vi "Begin.vi"() -> ()   [LabVIEW 2015]
doc: "Called before other user functions, this VI is expected to open initial I/O refnums, load in file data, and do all program initialization. Notice that the <B>error out</B> terminal is simply used for data flow. Wiring it to other structures or subVIs ensures that this VI runs first."
uses:
  <vilib>/Rock Robotics/WPI/DriverStation/WPI_DriverStationRobotMode2.ctl
  <vilib>/Rock Robotics/WPI/Joystick/WPI_JoystickDeviceEnum.ctl
  <vilib>/Rock Robotics/SystemInterfaces/DIO/FPGA_DIOChannel.ctl
  <vilib>/Rock Robotics/WPI/Encoder/WPI_EncoderType.ctl
  <vilib>/Rock Robotics/WPI/CAN/TalonSRX/WPI_CANTalonSRX_APIControlMode.ctl
  <vilib>/Rock Robotics/WPI/CAN/TalonSRX/WPI_CANTalonSRX_APIFeedbackSelect.ctl
  <vilib>/Rock Robotics/SystemInterfaces/DIO/FPGA_DIOPWMChannel.ctl
  Robot Global Data.vi
  <vilib>/Rock Robotics/Network Tables/NT Write String Array.vi
  <vilib>/Rock Robotics/WPI/Counter/WPI_CounterDigitalInputToDigitalSource.vi
  <vilib>/Rock Robotics/WPI/MotorControl/WPI_MotorControlOpenCANTalonSRX.vi
  <vilib>/Rock Robotics/WPI/MotorControl/WPI_MotorControlOpen VictorSP.vi
panel:
  in  "error in":errorcluster
  out "error out":errorcluster
  in  "I 3":dbl
  in  "F 3":dbl=0.01
  in  "D 3":dbl caption="D"
  in  "P 3":dbl=1.0 caption="P"
  in  "Reverse Feedback Sensor 3":bool
  in  "Slave Device Number 3":u8=1 caption="Slave Device Number"
  in  "Encoder Codes Per Rev 3":u16=360
  in  "Master Device Number 3":u8 caption="Master Device Number"
  in  "I 2":dbl
  in  "F 2":dbl=0.01
  in  "D 2":dbl caption="D"
  in  "P 2":dbl=1.0 caption="P"
  in  "Reverse Feedback Sensor 2":bool
  in  "Slave Device Number 2":u8=1 caption="Slave Device Number"
  in  "Encoder Codes Per Rev 2":u16=360
  in  "Master Device Number 2":u8 caption="Master Device Number"
  in  "I":dbl
  in  "F":dbl=0.01
  in  "D":dbl
  in  "P":dbl=1.0
  in  "Reverse Feedback Sensor":bool
  in  "Slave Device Number":u8=1
  in  "Encoder Codes Per Rev":u16=360
  in  "Master Device Number":u8
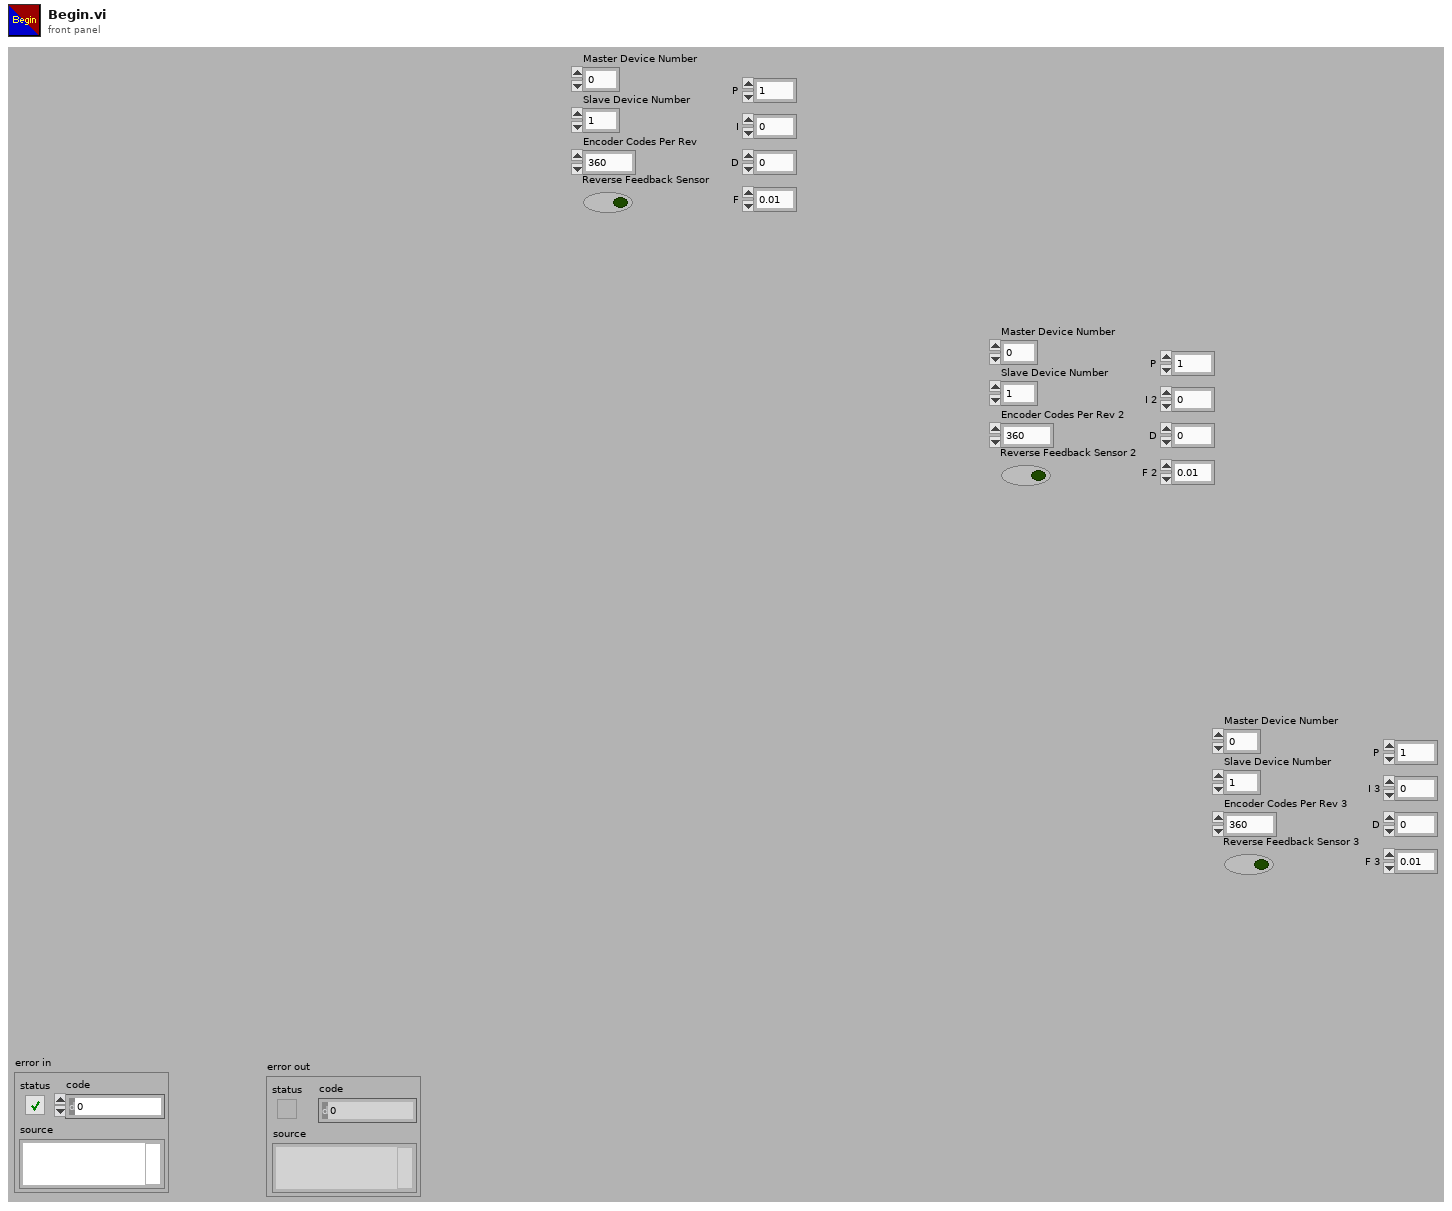
[diagram p1: front panel]
types:
  T1 = typedef "FPGA_DIOPWMChannel.ctl" = enum8{"PWM 0", "PWM 1", "PWM 2", "PWM 3", "PWM 4", "PWM 5", "PWM 6", "PWM 7", "PWM 8", "PWM 9", "PWM MXP 0", "PWM MXP 1", "PWM MXP 2", "PWM MXP 3", "PWM MXP 4", "PWM MXP 5", "PWM MXP 6", "PWM MXP 7", "PWM MXP 8", "PWM MXP 9", "Invalid"}
  T2 = typedef "WPI_EncoderType.ctl" = enum16{"1x", "2x", "4x"}
  T3 = typedef "FPGA_DIOChannel.ctl" = enum8{"DIO 0", "DIO 1", "DIO 2", "DIO 3", "DIO 4", "DIO 5", "DIO 6", "DIO 7", "DIO 8", "DIO 9", "DIO MXP 0", "DIO MXP 1", "DIO MXP 2", "DIO MXP 3", "DIO MXP 4", "DIO MXP 5", "DIO MXP 6", "DIO MXP 7", "DIO MXP 8", "DIO MXP 9", "DIO MXP 10", "DIO MXP 11", "DIO MXP 12", "DIO MXP 13", "DIO MXP 14", "DIO MXP 15", "Invalid"}
  T4 = typedef "WPI_JoystickDeviceEnum.ctl" = enum16{"USB 0", "USB 1", "USB 2", "USB 3", "USB 4", "USB 5"}
  T5 = typedef "WPI_CANTalonSRX_APIControlMode.ctl" = enum8{"Percent VBus", "Speed", "Position", "Slave", "Unchanged / Invalid", "Voltage Compensation", "Current", "Motion Profile"}
  T6 = typedef "WPI_CANTalonSRX_APIFeedbackSelect.ctl" = enum16{"Digital Quadrature Encoder", "Analog Potentiometer", "Analog Encoder", "Count on Quad-A (Rising-Edge)", "Count on Quad-A (Falling-Edge)", "CTR Magnetic Enc (Absolute)", "CTR Magnetic Enc (Relative)", "Pulse Width"}
  T7 = typedef "WPI_DriverStationRobotMode2.ctl" = enum16{"Autonomous Disabled", "Autonomous Enabled", "Teleop Disabled", "Teleop Enabled", "Disconnected", "Finish", "Test Disabled", "Test Enabled", "Emergency Stopped"}
  T8 = typedef "WPI_MotorControlDeviceRef.ctl" = cluster{"DeviceStatus":errorcluster, "Type":T9, "PWM":cluster{"PWM Channel":T1, "DeadBand":T10}, "CAN":cluster{"Device Number":u8, "Control Mode":T11, "Semaphore":T12, "Max Vout":dbl, "TalonSRX Control Mode":T5}, "Invert":bool}
  T9 = typedef "WPI_MotorControlType.ctl" = enum16{"PWM", "CAN", "CANTalonSRX"}
  T10 = typedef "WPI_PWMDeadband.ctl" = cluster{"Name":string, "maxPositivePwm":i32, "minPositivePwm":i32, "centerPwm":i32, "maxNegativePwm":i32, "minNegativePwm":i32, "angularRange":u16}
  T11 = typedef "WPI_CANJaguar_ControlMode.ctl" = enum8{"Percent VBus", "Current", "Speed", "Position", "Voltage"}
  T12 = typedef "Semaphore RefNum" = refnum<k1>
  T13 = typedef "WPI_JoystickDevRef.ctl" = cluster{"Device":T4}
  T14 = typedef "WPI_DigitalInputDevRef.ctl" = cluster{"DevStatus":errorcluster, "DIO Channel":T3}
  T15 = typedef "FPGA_CounterEncoderSourceConvertionLVSourceType.ctl" = cluster{"DevStatus":errorcluster, "AnalogTriggerMode?":bool, "DigitalMode":cluster{"DIO Channel":T16}, "AnalogTriggerMode":cluster{"AnalogTriggerIndex":T17, "OutputType":T18}}
  T16 = typedef "FPGA_DIODigitalSourceChannel.ctl" = enum8{"DIO 0", "DIO 1", "DIO 2", "DIO 3", "DIO 4", "DIO 5", "DIO 6", "DIO 7", "DIO 8", "DIO 9", "DIO MXP 0", "DIO MXP 1", "DIO MXP 2", "DIO MXP 3", "DIO MXP 4", "DIO MXP 5", "DIO MXP 6", "DIO MXP 7", "DIO MXP 8", "DIO MXP 9", "DIO MXP 10", "DIO MXP 11", "DIO MXP 12", "DIO MXP 13", "DIO MXP 14", "DIO MXP 15", "Disabled"}
  T17 = typedef "FPGA_AnalogTriggerIndex.ctl" = enum8{"Trig 0", "Trig 1", "Trig 2", "Trig 3", "Trig 4", "Trig 5", "Trig 6", "Trig 7", "Invalid"}
  T18 = typedef "FPGA_AnalogTriggerOutType.ctl" = enum16{"InWindow", "TriggerState", "Rising", "Falling"}
  T19 = typedef "WPI_EncoderDevRef.ctl" = cluster{"DevStatus":errorcluster, "EncoderIndex":T20, "CounterIndex":T21, "DistancePerCount":dbl, "Decoding Type":T2}
  T20 = typedef "FPGA_EncoderIdx.ctl" = enum8{"Enc 0", "Enc 1", "Enc 2", "Enc 3", "Enc 4", "Enc 5", "Enc 6", "Enc 7", "Invalid"}
  T21 = typedef "FPGA_CounterCtrSystemIndex.ctl" = enum8{"Ctr 0", "Ctr 1", "Ctr 2", "Ctr 3", "Ctr 4", "Ctr 5", "Ctr 6", "Ctr 7", "Invalid"}
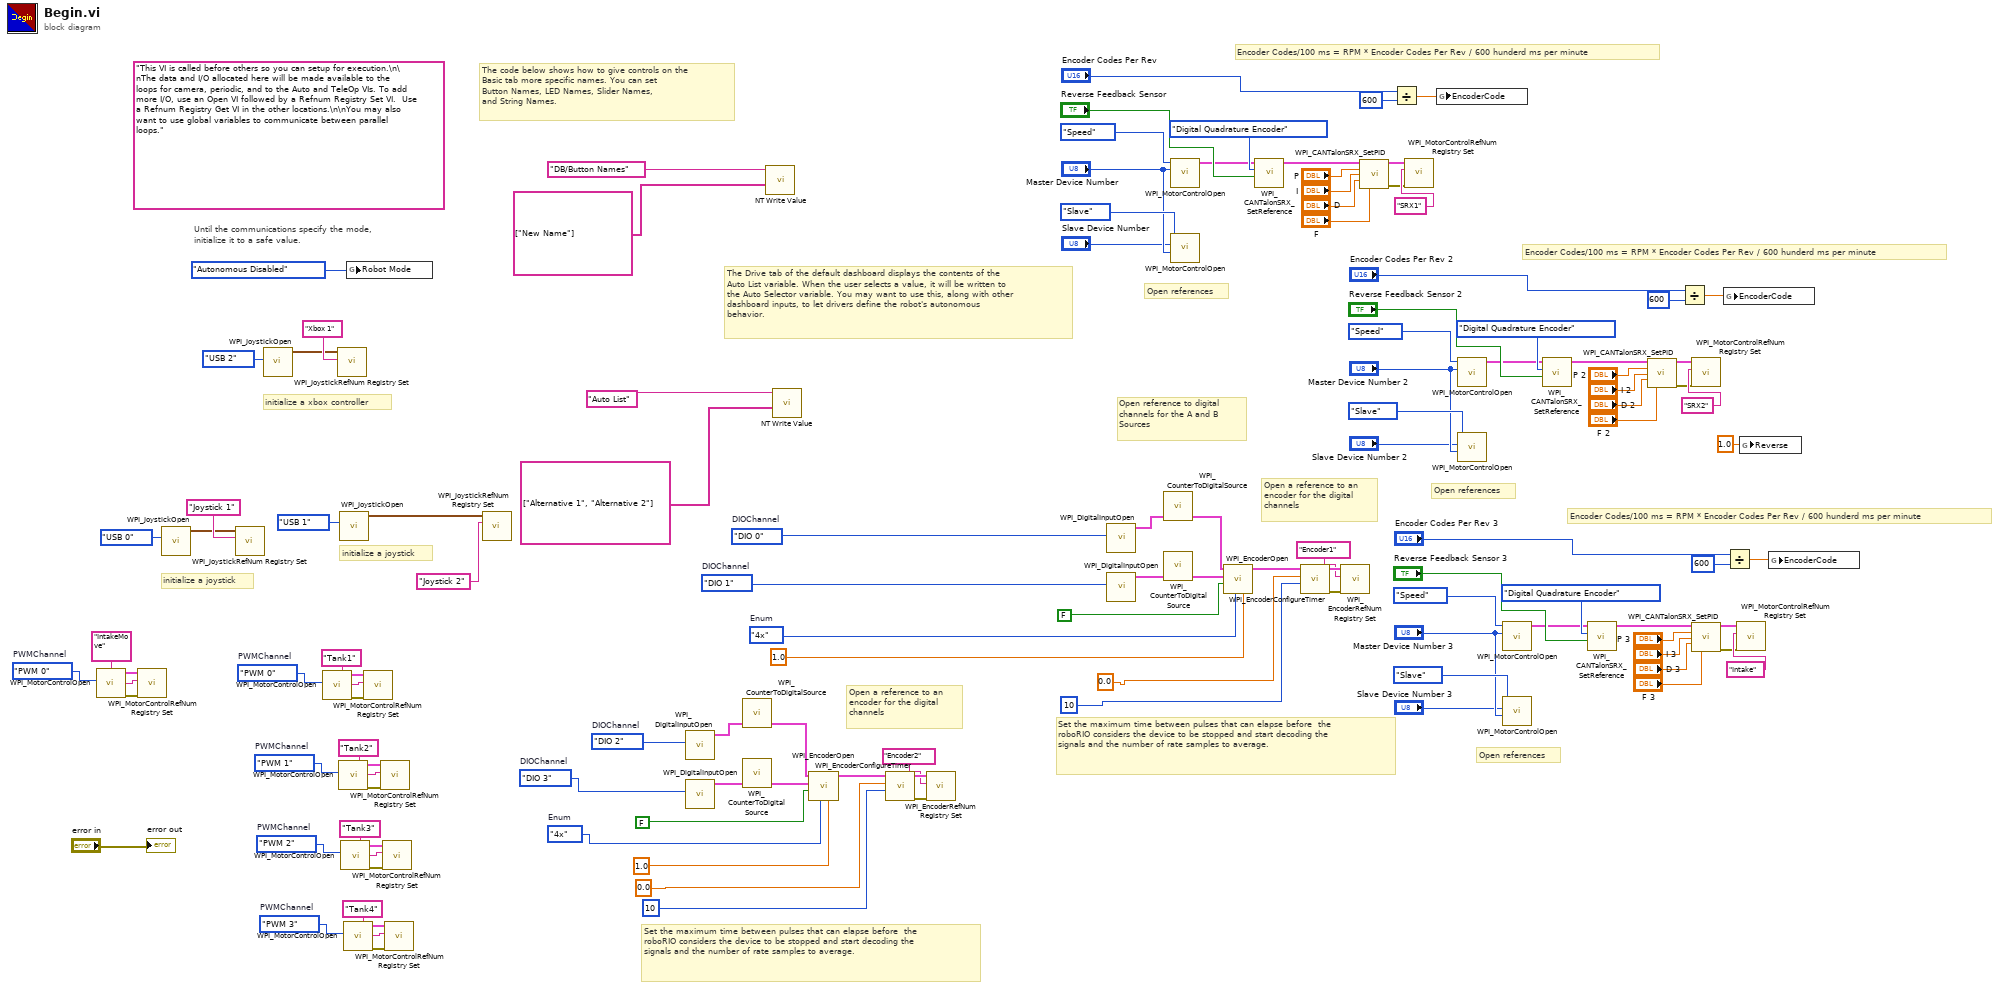
[diagram p0: block diagram]
diagram:
  w2 = FPGA_DIOPWMChannel."PWM 0"  # PWMChannel
  w6 = FPGA_DIOPWMChannel."PWM 3"  # PWMChannel
  w10 = FPGA_DIOPWMChannel."PWM 2"  # PWMChannel
  w14 = FPGA_DIOPWMChannel."PWM 1"  # PWMChannel
  w18 = FPGA_DIOPWMChannel."PWM 0"  # PWMChannel
  w26 = WPI_EncoderType."4x"  # Enum
  w28 = FPGA_DIOChannel."DIO 3"  # DIOChannel
  w29 = FPGA_DIOChannel."DIO 2"  # DIOChannel
  w98 = WPI_EncoderType."4x"  # Enum
  w100 = FPGA_DIOChannel."DIO 1"  # DIOChannel
  w101 = FPGA_DIOChannel."DIO 0"  # DIOChannel
  (unwired) "This VI is called before others so you can setup for execution.\n\nThe data and I/O allocated here will be made available to the loops for camera, periodic, and to the Auto and TeleOp VIs. To add more I/O, use an Open VI followed by a Refnum Registry Set VI.  Use a Refnum Registry Get VI in the other locations.\n\nYou may also want to use global variables to communicate between parallel loops."
  # "Set the maximum time between pulses that can elapse before  the roboRIO considers the device to be stopped and start decoding the signals and the number of rate samples to average."
  # "Open a reference to an\nencoder for the digital \nchannels"
  # "initialize a xbox controller"
  # "Encoder Codes/100 ms = RPM * Encoder Codes Per Rev / 600 hunderd ms per minute"
  # "Open references"
  # "Encoder Codes/100 ms = RPM * Encoder Codes Per Rev / 600 hunderd ms per minute"
  # "Open references"
  # "Encoder Codes/100 ms = RPM * Encoder Codes Per Rev / 600 hunderd ms per minute"
  # "Open references"
  # "The Drive tab of the default dashboard displays the contents of the\nAuto List variable. When the user selects a value, it will be written to\nthe Auto Selector variable. You may want to use this, along with other\ndashboard inputs, to let drivers define the robot's autonomous\nbehavior."
  # "Set the maximum time between pulses that can elapse before  the roboRIO considers the device to be stopped and start decoding the signals and the number of rate samples to average."
  # "Open a reference to an\nencoder for the digital \nchannels"
  # "Open reference to digital \nchannels for the A and B\nSources"
  # "initialize a joystick"
  # "initialize a joystick"
  # "The code below shows how to give controls on the\nBasic tab more specific names. You can set\nButton Names, LED Names, Slider Names,\nand String Names."
  # "Until the communications specify the mode,\ninitialize it to a safe value."
  n1 = call-poly <vilib>:"WPI_MotorControlOpen.vi"("PWM Channel"=w2) -> ("error out"=w5:errorcluster, "MotorControlDeviceRef"=w4:T8)  [unwired: 9 in]
  n2 = call <vilib>:"WPI_MotorControlRefNum Registry Set.vi"("error in (no error)"=w5, "refnum name"="IntakeMove", "MotorControlDevRef"=w4) -> ()  [unwired: 7 in, 2 out]
  n3 = call <vilib>:"WPI_JoystickOpen.vi"("JoystickDevice"=WPI_JoystickDeviceEnum."USB 0") -> ("JoystickDevRef"=w114:T13)  [unwired: 10 in]
  n4 = call <vilib>:"WPI_JoystickRefNum Registry Set.vi"("refnum name"="Joystick 1", "JoystickDevRef"=w114) -> ()  [unwired: 8 in, 2 out]
  n5 = call <vilib>:"WPI_JoystickOpen.vi"("JoystickDevice"=WPI_JoystickDeviceEnum."USB 2") -> ("JoystickDevRef"=w39:T13)  [unwired: 10 in]
  n6 = call-poly <vilib>:"WPI_MotorControlOpen.vi"("PWM Channel"=w18) -> ("error out"=w21:errorcluster, "MotorControlDeviceRef"=w20:T8)  [unwired: 9 in]
  n7 = call <vilib>:"WPI_JoystickRefNum Registry Set.vi"("refnum name"="Xbox 1", "JoystickDevRef"=w39) -> ()  [unwired: 8 in, 2 out]
  n8 = call-poly <vilib>:"WPI_MotorControlOpen.vi"("PWM Channel"=w14) -> ("error out"=w17:errorcluster, "MotorControlDeviceRef"=w16:T8)  [unwired: 9 in]
  n9 = call <vilib>:"WPI_JoystickOpen.vi"("JoystickDevice"=WPI_JoystickDeviceEnum."USB 1") -> ("JoystickDevRef"=w111:T13)  [unwired: 10 in]
  n10 = call-poly <vilib>:"WPI_MotorControlOpen.vi"("PWM Channel"=w10) -> ("error out"=w13:errorcluster, "MotorControlDeviceRef"=w12:T8)  [unwired: 9 in]
  n11 = call-poly <vilib>:"WPI_MotorControlOpen.vi"("PWM Channel"=w6) -> ("error out"=w9:errorcluster, "MotorControlDeviceRef"=w8:T8)  [unwired: 9 in]
  n12 = global write "Robot Global Data.vi" "Robot Mode"(WPI_DriverStationRobotMode2."Autonomous Disabled" ("Robot Mode")) -> ()
  n13 = call <vilib>:"WPI_MotorControlRefNum Registry Set.vi"("error in (no error)"=w21, "refnum name"="Tank1", "MotorControlDevRef"=w20) -> ()  [unwired: 7 in, 2 out]
  n14 = call <vilib>:"WPI_MotorControlRefNum Registry Set.vi"("error in (no error)"=w17, "refnum name"="Tank2", "MotorControlDevRef"=w16) -> ()  [unwired: 7 in, 2 out]
  n15 = call <vilib>:"WPI_MotorControlRefNum Registry Set.vi"("error in (no error)"=w13, "refnum name"="Tank3", "MotorControlDevRef"=w12) -> ()  [unwired: 7 in, 2 out]
  n16 = call <vilib>:"WPI_MotorControlRefNum Registry Set.vi"("error in (no error)"=w9, "refnum name"="Tank4", "MotorControlDevRef"=w8) -> ()  [unwired: 7 in, 2 out]
  n17 = call <vilib>:"WPI_JoystickRefNum Registry Set.vi"("refnum name"="Joystick 2", "JoystickDevRef"=w111) -> ()  [unwired: 8 in, 2 out]
  n18 = call <vilib>:"WPI_DigitalInputOpen.vi"("DIO Channel"=w29) -> ("DigitalInputDevRef"=w35:T14)  [unwired: 1 in, 9 out]
  n19 = call <vilib>:"WPI_DigitalInputOpen.vi"("DIO Channel"=w28) -> ("DigitalInputDevRef"=w36:T14)  [unwired: 1 in, 9 out]
  n20 = call-poly <vilib>:"WPI_CounterToDigitalSource.vi"("DigitalInputDevRef"=w35) -> ("Digital Source"=w34:T15)  [unwired: 6 out]
  n21 = call-poly <vilib>:"WPI_CounterToDigitalSource.vi"("DigitalInputDevRef"=w36) -> ("Digital Source"=w37:T15)  [unwired: 6 out]
  n22 = call-poly <vilib>:"NT Write Value.vi"("String Array"=string[] ["New Name"], "Name"="DB/Button Names") -> ()  [unwired: 9 in, 1 out]
  n23 = call-poly <vilib>:"NT Write Value.vi"("String Array"=string[] ["Alternative 1", "Alternative 2"], "Name"="Auto List") -> ()  [unwired: 9 in, 1 out]
  n24 = call <vilib>:"WPI_EncoderOpen.vi"("DistancePerCount"=1.0, "Decoding Type"=w26, "Invert Direction (False)"=FALSE, "BSource"=w37, "ASource"=w34) -> ("EncoderDevRef"=w33:T19)  [unwired: 3 in, 3 out]
  n25 = call <vilib>:"WPI_EncoderConfigureTimer.vi"("Number Samples to Average"=10, "Minimum Rate"=0.0, "EncoderDevRef"=w33) -> ("error out"=w32:errorcluster, "EncoderDevRef"=w31:T19)  [unwired: 1 in, 6 out]
  n26 = call <vilib>:"WPI_EncoderRefNum Registry Set.vi"("error in (no error)"=w32, "refnum name"="Encoder2", "EncoderDevRef"=w31) -> ()  [unwired: 7 in, 2 out]
  n27 = call <vilib>:"WPI_DigitalInputOpen.vi"("DIO Channel"=w101) -> ("DigitalInputDevRef"=w107:T14)  [unwired: 1 in, 9 out]
  n28 = call <vilib>:"WPI_DigitalInputOpen.vi"("DIO Channel"=w100) -> ("DigitalInputDevRef"=w108:T14)  [unwired: 1 in, 9 out]
  n29 = call-poly <vilib>:"WPI_CounterToDigitalSource.vi"("DigitalInputDevRef"=w107) -> ("Digital Source"=w106:T15)  [unwired: 6 out]
  n30 = call-poly <vilib>:"WPI_CounterToDigitalSource.vi"("DigitalInputDevRef"=w108) -> ("Digital Source"=w109:T15)  [unwired: 6 out]
  n31 = call-poly <vilib>:"WPI_MotorControlOpen.vi"("Device Number"="Master Device Number", "Control Mode"=WPI_CANTalonSRX_APIControlMode."Speed") -> ("MotorControlDeviceRef"=w84:T8)  [unwired: 3 in, 6 out]
  n32 = call-poly <vilib>:"WPI_MotorControlOpen.vi"("Master Device Number"="Master Device Number", "Device Number"="Slave Device Number", "Control Mode"=WPI_CANTalonSRX_APIControlMode."Slave") -> ()  [unwired: 2 in, 7 out]
  n33 = call <vilib>:"WPI_EncoderOpen.vi"("DistancePerCount"=1.0, "Decoding Type"=w98, "Invert Direction (False)"=FALSE, "BSource"=w109, "ASource"=w106) -> ("EncoderDevRef"=w105:T19)  [unwired: 3 in, 3 out]
  n34 = call <vilib>:"WPI_CANTalonSRX_SetReference.vi"("Reverse Feedback Sensor"="Reverse Feedback Sensor", "Feedback Reference"=WPI_CANTalonSRX_APIFeedbackSelect."Digital Quadrature Encoder", "CAN Talon SRX Ref"=w84) -> ("CAN Talon SRX Ref"=w83:T8)  [unwired: 7 in, 1 out]
  n35 = call <vilib>:"WPI_EncoderConfigureTimer.vi"("Number Samples to Average"=10, "Minimum Rate"=0.0, "EncoderDevRef"=w105) -> ("error out"=w104:errorcluster, "EncoderDevRef"=w103:T19)  [unwired: 1 in, 6 out]
  n36 = call <vilib>:"WPI_EncoderRefNum Registry Set.vi"("error in (no error)"=w104, "refnum name"="Encoder1", "EncoderDevRef"=w103) -> ()  [unwired: 7 in, 2 out]
  n37 = call <vilib>:"WPI_CANTalonSRX_SetPID.vi"("CAN Talon SRX Ref"=w83, "P"="P", "I"="I", "D"="D", "F"="F") -> ("CAN Talon SRX Ref"=w79:T8, "error out"=w77:errorcluster)  [unwired: 9 in]
  n38 = Divide(x="Encoder Codes Per Rev", y=u16 600) -> (x/y=w80:dbl)
  n39 = call <vilib>:"WPI_MotorControlRefNum Registry Set.vi"("error in (no error)"=w77, "refnum name"="SRX1", "MotorControlDevRef"=w79) -> ()  [unwired: 7 in, 2 out]
  n40 = global write "Robot Global Data.vi" "EncoderCode"(w80) -> ()
  n41 = call-poly <vilib>:"WPI_MotorControlOpen.vi"("Device Number"="Master Device Number 2", "Control Mode"=WPI_CANTalonSRX_APIControlMode."Speed") -> ("MotorControlDeviceRef"=w66:T8)  [unwired: 3 in, 6 out]
  n42 = call-poly <vilib>:"WPI_MotorControlOpen.vi"("Master Device Number"="Master Device Number 2", "Device Number"="Slave Device Number 2", "Control Mode"=WPI_CANTalonSRX_APIControlMode."Slave") -> ()  [unwired: 2 in, 7 out]
  n43 = call-poly <vilib>:"WPI_MotorControlOpen.vi"("Device Number"="Master Device Number 3", "Control Mode"=WPI_CANTalonSRX_APIControlMode."Speed") -> ("MotorControlDeviceRef"=w48:T8)  [unwired: 3 in, 6 out]
  n44 = call-poly <vilib>:"WPI_MotorControlOpen.vi"("Master Device Number"="Master Device Number 3", "Device Number"="Slave Device Number 3", "Control Mode"=WPI_CANTalonSRX_APIControlMode."Slave") -> ()  [unwired: 2 in, 7 out]
  n45 = call <vilib>:"WPI_CANTalonSRX_SetReference.vi"("Reverse Feedback Sensor"="Reverse Feedback Sensor 2", "Feedback Reference"=WPI_CANTalonSRX_APIFeedbackSelect."Digital Quadrature Encoder", "CAN Talon SRX Ref"=w66) -> ("CAN Talon SRX Ref"=w65:T8)  [unwired: 7 in, 1 out]
  n46 = call <vilib>:"WPI_CANTalonSRX_SetReference.vi"("Reverse Feedback Sensor"="Reverse Feedback Sensor 3", "Feedback Reference"=WPI_CANTalonSRX_APIFeedbackSelect."Digital Quadrature Encoder", "CAN Talon SRX Ref"=w48) -> ("CAN Talon SRX Ref"=w47:T8)  [unwired: 7 in, 1 out]
  n47 = call <vilib>:"WPI_CANTalonSRX_SetPID.vi"("CAN Talon SRX Ref"=w65, "P"="P 2", "I"="I 2", "D"="D 2", "F"="F 2") -> ("CAN Talon SRX Ref"=w61:T8, "error out"=w59:errorcluster)  [unwired: 9 in]
  n48 = Divide(x="Encoder Codes Per Rev 2", y=u16 600) -> (x/y=w62:dbl)
  n49 = call <vilib>:"WPI_MotorControlRefNum Registry Set.vi"("error in (no error)"=w59, "refnum name"="SRX2", "MotorControlDevRef"=w61) -> ()  [unwired: 7 in, 2 out]
  n50 = call <vilib>:"WPI_CANTalonSRX_SetPID.vi"("CAN Talon SRX Ref"=w47, "P"="P 3", "I"="I 3", "D"="D 3", "F"="F 3") -> ("CAN Talon SRX Ref"=w43:T8, "error out"=w41:errorcluster)  [unwired: 9 in]
  n51 = global write "Robot Global Data.vi" "EncoderCode"(w62) -> ()
  n52 = Divide(x="Encoder Codes Per Rev 3", y=u16 600) -> (x/y=w44:dbl)
  n53 = call <vilib>:"WPI_MotorControlRefNum Registry Set.vi"("error in (no error)"=w41, "refnum name"="Intake", "MotorControlDevRef"=w43) -> ()  [unwired: 7 in, 2 out]
  n54 = global write "Robot Global Data.vi" "Reverse"(1.0) -> ()
  n55 = global write "Robot Global Data.vi" "EncoderCode"(w44) -> ()
  "error out" <- "error in"
